vi "Bind Named Numeric Strings.vi"(8 "error in (no error)":errorcluster, 9 "Datum Name (\"\"=Use Control Label)":string, 10 "NmdNum Refnum":refnum<vi>, 11 "IViewable in":refnum<class "IViewable.lvclass">) -> (0 "error out":errorcluster, 3 "IViewable out":refnum<class "IViewable.lvclass">)   [LabVIEW 2015, in "IViewable.lvlib" / "IViewable.lvclass"]
doc: "Bind the Strings of a NamedNumeric control terminal to a published 1-D array of strings."
uses:
  IViewable.lvclass
  <vilib>/ActorFramework/Actor/Actor.lvclass/Actor.ctl
  <vilib>/ActorFramework/Message Enqueuer/Message Enqueuer.lvclass/Message Enqueuer.ctl
  Transport/NamedNumericStringsBinding/NamedNumericStringsBinding.lvclass/NamedNumericStringsBinding.ctl
  SubscriptionPolicy/ValueChangeSubscription/ValueChangeSubscription.lvclass/ValueChangeSubscription.ctl
  IMediator/SubscriptionRequest/SubscriptionRequest.lvclass/SubscriptionRequest.ctl
  IObserver/IObserver Messages/Subscribe Msg/Subscribe Msg.lvclass/Subscribe Msg.ctl
  <vilib>/ActorFramework/Message Enqueuer/Init from Existing Queue.vi
  <vilib>/ActorFramework/Message Enqueuer/Enqueue.vi
  <vilib>/ActorFramework/Message Priority Queue/Priority Enqueue.vi
  SubscriptionPolicy/ValueChangeSubscription/ValueChangeSubscription.lvclass
  <vilib>/ActorFramework/Message Enqueuer/Message Enqueuer.lvclass
  Transport/NamedNumericStringsBinding/NamedNumericStringsBinding.lvclass
  IMediator/SubscriptionRequest/SubscriptionRequest.lvclass
  IObserver/IObserver Messages/Subscribe Msg/Subscribe Msg.lvclass
  IObserver/IObserver/IObserver.lvclass
  <vilib>/ActorFramework/Actor/Actor.lvclass
  IMediator/ISubscriptionPolicy/ISubscriptionPolicy.lvclass
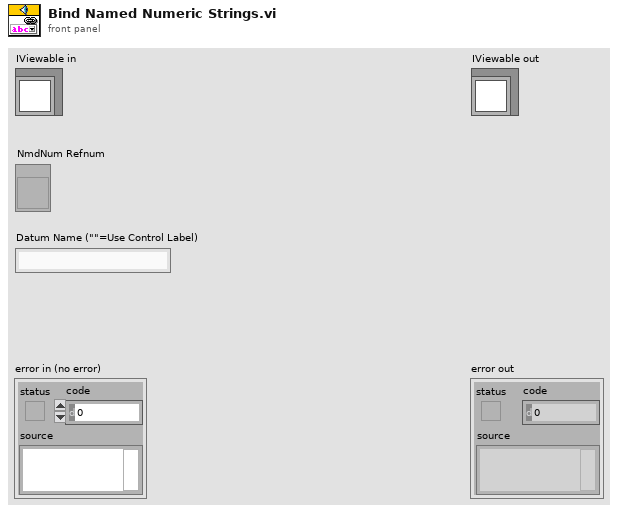
[diagram p1: front panel]
types:
  T1 = typedef "IMediator.lvlib/ISubscriptionPolicy.lvclass/ISubscriptionPolicy Reference.ctl" = refnum<data-value>
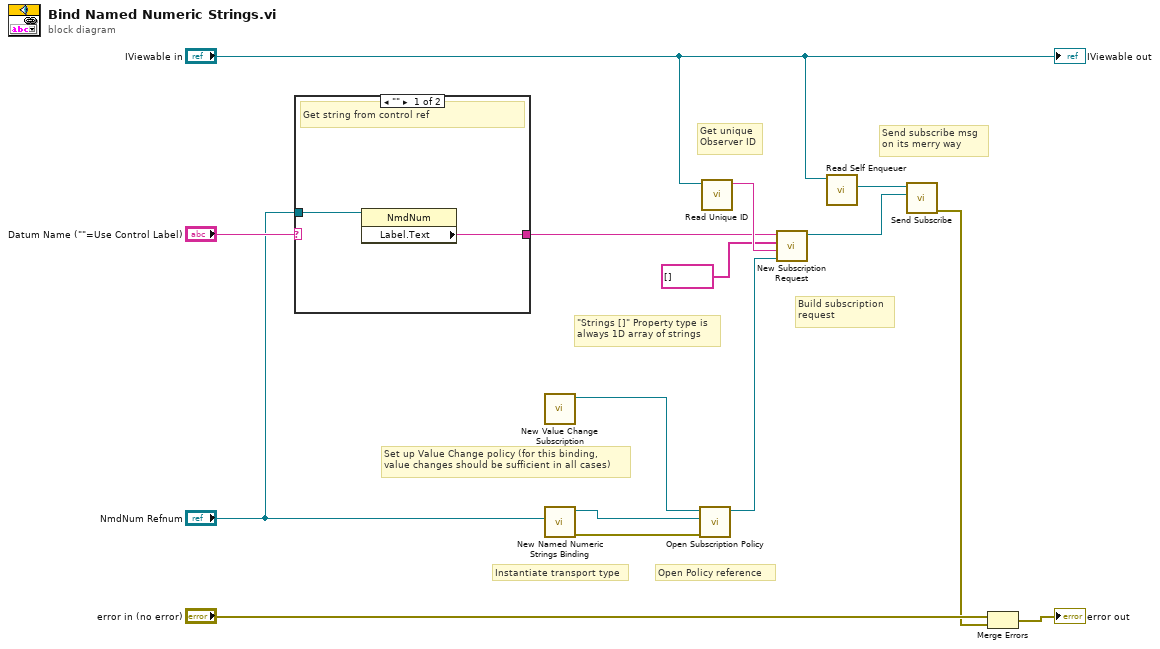
[diagram p0: block diagram]
diagram:
  # "\"Strings []\" Property type is\nalways 1D array of strings"
  # "Open Policy reference"
  # "Set up Value Change policy (for this binding,\nvalue changes should be sufficient in all cases)"
  # "Send subscribe msg\non its merry way"
  # "Build subscription\nrequest"
  # "Get unique\nObserver ID"
  # "Instantiate transport type"
  n1 = case shown="\"\"" "Datum Name (\"\"=Use Control Label)" {
    selector: "Datum Name (\"\"=Use Control Label)" -> [_ w18]
    tunnel: [w16 w18] -> w8
    tunnel: "NmdNum Refnum" -> [w17 _]
    frame "" {
      # "Get string from control ref"
      n2 = property class="NmdNum"(reference=w17) -> ("Label.Text"=w16:string)  [unwired: 1 in, 2 out]
    }
    frame Default {
      # "Use string wired to input terminal"
    }
  }
  n3 = call "New Value Change Subscription.vi"() -> ("ValueChangeSubscription Out"=w3:refnum<class "ValueChangeSubscription.lvclass">)  [unwired: 11 in]
  n4 = call "New Named Numeric Strings Binding.vi"("NmdNum Refnum"="NmdNum Refnum") -> ("error out"=w2:errorcluster, "NamedNumericStringsBinding"=w5:refnum<class "NamedNumericStringsBinding.lvclass">)  [unwired: 9 in]
  n5 = call "Open Subscription Policy.vi"("error in (no error)"=w2, "Transport"=w5, "SubscriptionPolicy"=w3) -> ("Subscription Policy"=w6:T1)  [unwired: 7 in, 1 out]
  n6 = call "Read Unique ID.vi"("IObserver In"="IViewable in") -> ("Unique ID"=w14:string)  [unwired: 10 in]
  n7 = call "New Subscription Request.vi"("Subscription Policy"=w6, "Subscriber ID"=w14, "Type"=string[] [], "Datum Name"=w8) -> ("SubscriptionRequest"=w4:refnum<class "SubscriptionRequest.lvclass">)  [unwired: 7 in]
  n8 = call <vilib>:"Read Self Enqueuer.vi"("Actor"="IViewable in") -> ("Self Enqueuer"=w12:refnum<class "Message Enqueuer.lvclass">)  [unwired: 10 in]
  n9 = call "Send Subscribe.vi"("SubscriptionRequest"=w4, "Message Enqueuer"=w12) -> ("error out"=w10:errorcluster)  [unwired: 8 in, 1 out]
  n10 = Merge Errors("error in (no error)", w10) -> (→"error out":errorcluster)
  "IViewable out" <- "IViewable in"
